vi "decodeStream.vi"(8 "error in (no error)":errorcluster, 9 "beginIndex":i32, 10 "binary stream":u8[](array[numeric]), 11 "tBSON_I32 in":refnum<class "tBSON_I32.lvclass">) -> (0 "error out":errorcluster, 1 "endIndex":i32, 2 "binary stream out":u8[](array[numeric]), 3 "tBSON_I32 out":refnum<class "tBSON_I32.lvclass">)   [LabVIEW 2013, in "BSON.lvlib" / "tBSON_I32.lvclass"]
uses:
  tBSON_I32.lvclass
  tBSONElement/tBSONElement.lvclass
  setValue.vi
  BSON.lvlib
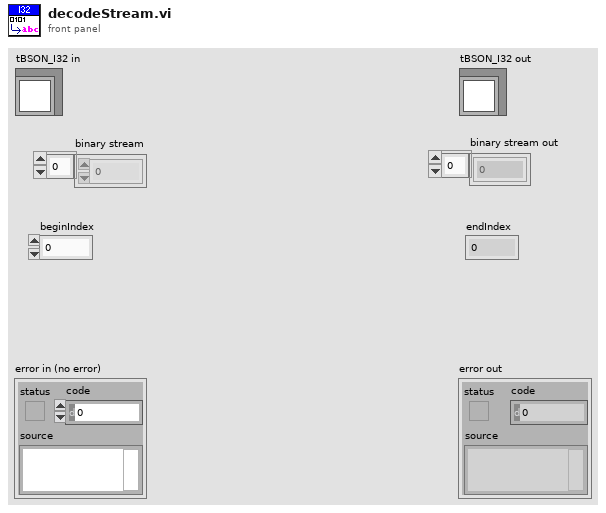
[diagram p1: front panel]
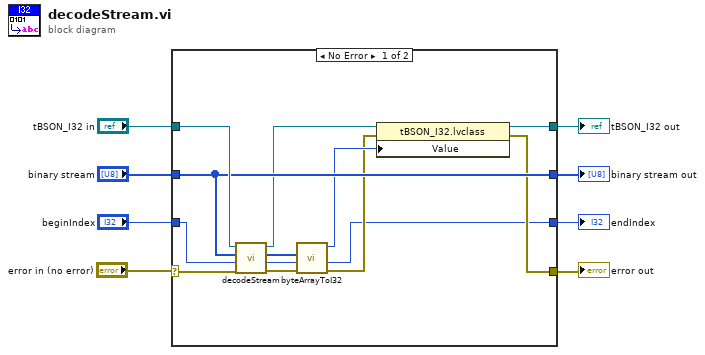
[diagram p0: block diagram]
diagram:
  n1 = case shown="No Error" "error in (no error)" {
    selector: "error in (no error)" -> [w21 w25]
    tunnel: [w15 w25] -> w7
    tunnel: "beginIndex" -> [w19 w24]
    tunnel: [w9 w24] -> w5
    tunnel: "binary stream" -> [w18 w23]
    tunnel: [w18 w23] -> w3
    tunnel: "tBSON_I32 in" -> [w20 w22]
    tunnel: [w14 w22] -> w1
    frame No Error {
      n2 = call-parent "decodeStream.vi"("error in (no error)"=w21, "beginIndex"=w19, "binary stream"=w18, "tBSONElement in"=w20) -> ("error out"=w13:errorcluster, "endIndex"=w10:i32, "binary stream out"=w11:u8[], "tBSONElement out"=w17:refnum<class "tBSON_I32.lvclass">)  [unwired: 4 in]
      n3 = call "byteArrayToI32.vi"("error in (no error)"=w13, "StartIndex"=w10, "ByteArrayIn"=w11) -> ("error out"=w12:errorcluster, "EndIndex"=w9:i32, "I32"=w16:i32)  [unwired: 5 in, 1 out]
      n4 = property class="tBSON_I32.lvclass"(reference=w17, error in=w12, "Value"=w16) -> (reference out=w14:refnum<class "tBSON_I32.lvclass">, error out=w15:errorcluster)
    }
    frame Error {
    }
  }
  "error out" <- w7
  "tBSON_I32 out" <- w1
  "binary stream out" <- w3
  "endIndex" <- w5
